vi "Get Run for Execution.vi"(8 "error in (no error)":errorcluster, 11 "Optimiser Cell in":refnum<class "Optimiser Cell.lvclass">) -> (0 "error out":errorcluster, 1 "Last Script":bool, 2 "Run Instance":refnum<class "Run Instance.lvclass">, 3 "Optimiser Cell out":refnum<class "Optimiser Cell.lvclass">)   [LabVIEW 2020, in "CIRCUS_uServices.lvlib" / "Run Utilities.lvlib" / "Optimiser Cell.lvclass"]
doc: "Get Run Instance from the Cell and change the status of the Cell to active. This VI is for manipulating Runs from the Schedule and shouldn't be used just to access the Run Instance. For obtaining Run Instance use the Read functions from Accessors or through the property node"
uses:
  Optimiser Cell.lvclass
  Optimiser Cell.lvclass/Optimiser Cell.ctl
  Run Instance/Run Instance.lvclass
  Cell/Schedule Cell.lvclass
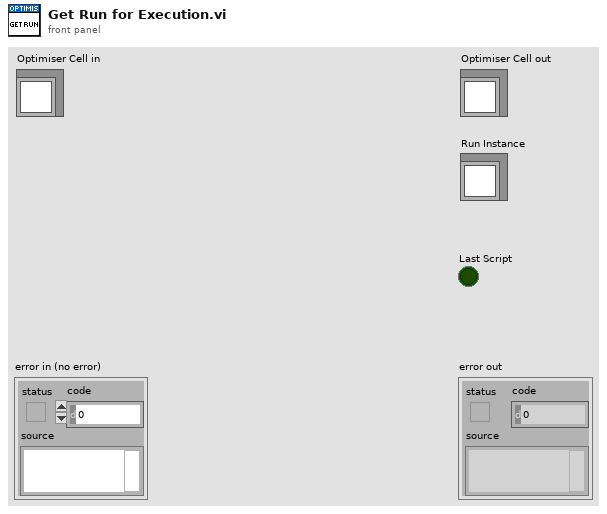
[diagram p1: front panel]
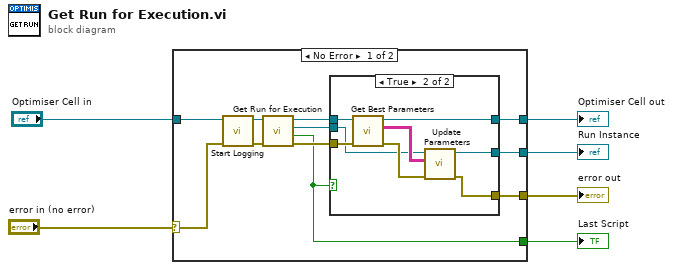
[diagram p0: block diagram]
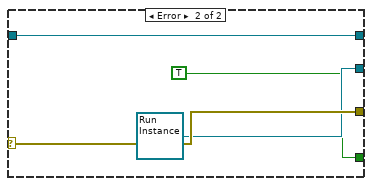
[diagram p3: hidden frame]
diagram:
  n1 = case shown="No Error" "error in (no error)" {
    selector: "error in (no error)" -> [w7 w32]
    tunnel: [w15 w32] -> w4
    tunnel: [w10 w31] -> w3
    tunnel: "Optimiser Cell in" -> [w8 w31]
    tunnel: [w16 refnum<class "Run Instance.lvclass"> refnum ("Run Instance")] -> w2
    tunnel: [w9 TRUE ("Last Script")] -> w1
    frame No Error {
      n2 = call-dynamic "Start Logging.vi"("error in (no error)"=w7, "Optimiser Cell in"=w8) -> ("error out"=w12:errorcluster, "Optimiser Cell out"=w13:refnum<class "Optimiser Cell.lvclass">)  [unwired: 8 in]
      n3 = call-parent "Get Run for Execution.vi"("error in (no error)"=w12, "Schedule Cell in"=w13) -> ("error out"=w17:errorcluster, "Last Script"=w9:bool, "Run Instance"=w14:refnum<class "Run Instance.lvclass">, "Schedule Cell out"=w11:refnum<class "Optimiser Cell.lvclass">)  [unwired: 6 in]
      n4 = case shown="True" w9 {
        tunnel: [w19 w26] -> w16
        tunnel: w17 -> [w20 w24]
        tunnel: [w20 w25] -> w15
        tunnel: w14 -> [w19 w22]
        tunnel: w11 -> [w18 w23]
        tunnel: [w18 w21] -> w10
        frame False {
        }
        frame True {
          n5 = call-dynamic "Get Best Parameters.vi"("error in (no error)"=w24, "Run Optimiser in"=w23) -> ("error out"=w28:errorcluster, "Best Parameters"=w27:string[][], "Run Optimiser out"=w21:refnum<class "Optimiser Cell.lvclass">)  [unwired: 7 in]
          n6 = call-dynamic "Update Parameters.vi"("error in (no error)"=w28, "Parameters"=w27, "Run Instance in"=w22) -> ("error out"=w25:errorcluster, "Run Instance out"=w26:refnum<class "Run Instance.lvclass">)  [unwired: 6 in, 1 out]
        }
      }
    }
    frame Error {
    }
  }
  "error out" <- w4
  "Optimiser Cell out" <- w3
  "Run Instance" <- w2
  "Last Script" <- w1
